vi "[FPGA] FXPT SawtoothGen Basic (use inside SCTL).vi"(7 "reset (rising edge)":bool, 11 "Carrier Frequency (=fo(Hz)*2*dT)":fxp<+/-,32,1>=0.0010350001975893974) -> (3 "Sawtooth":fxp<+/-,32,1> format="%.32g")   [LabVIEW 2015]
doc: "This VI generates the next point on a DDS generated sine wave.\n\nThe accumulator increments to calculate the next phase value in the waveform. By varying the accumulator increment you control the frequency of the sine wave.\n\nThe accumulator phase value is used to select a value from the sine wave reference waveform stored in the Lookup Table VI. The waveformcan be p[hase shifted by specifying a non-zero phase shift value which is added to the accumulator phase. The output from the LUT is scaled using the AO Amplitude value."
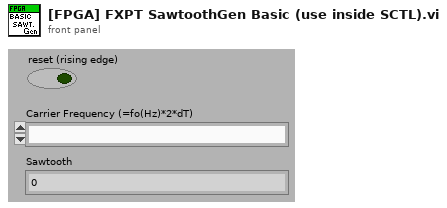
[diagram p1: front panel]
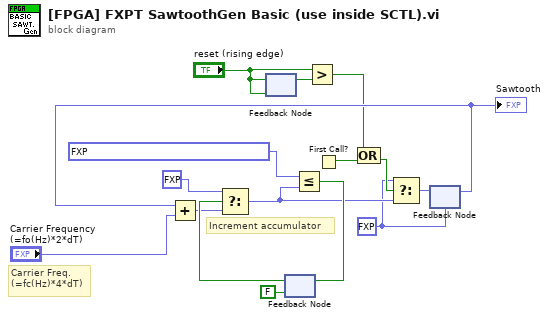
[diagram p0: block diagram]
diagram:
  w5 = fxp<+/-,32,1> 0.0 ("x+y")
  # "Carrier Freq. \n(=fc(Hz)*4*dT)"
  # "Increment accumulator"
  n1 = feedback #1("reset (rising edge)") -> (w4:bool)
  n2 = feedback-in #1("reset (rising edge)") -> ()
  n3 = feedback #2(FALSE) -> (w15:bool)
  n4 = Greater?(x="reset (rising edge)", y=w4) -> (0:w2:bool)
  n5 = First Call?() -> (First Call?: T/F=w1:bool)
  n6 = Compound Arithmetic op=OR(w2, w1) -> (w12:bool)
  n7 = feedback #3(w5) -> (w13:fxp<+/-,32,1>)
  "Sawtooth" <- w13
  n8 = Add(x=w13, y="Carrier Frequency (=fo(Hz)*2*dT)") -> (x+y=w9:fxp<+/-,32,1>)
  n9 = Select(t=fxp<+/-,32,1> -1.0 ("x+y"), s=w15, f=w9) -> (s? t:f=w6:fxp<+/-,32,1>)
  n10 = Less Or Equal?(x=fxp<+/-,32,1> 0.9999999995343387 ("x+y"), y=w6) -> (x <= y?=w7:bool)
  n11 = feedback-in #2(w7) -> ()
  n12 = Select(t=w5, s=w12, f=w6) -> (s? t:f=w14:fxp<+/-,32,1>)
  n13 = feedback-in #3(w14) -> ()
